vi "Model - DeInit.vi"(8 "error in (no error)":errorcluster, 11 "View Model":T1) -> (0 "error out":errorcluster)   [LabVIEW 2017]
doc: "De - initialize View Model"
uses:
  Controls/View Model.ctl
  Error Handler/Controls/Error Model.ctl
  Error Handler/Controls/Error Type.ctl
  Controls/Shared Model.ctl
  Elevator Controller/Controls/Elevator Model.ctl
  Elevator Controller/Controls/Controller Overhead.ctl
  Elevator Controller/Controls/Elevator Commands.ctl
  Configuration/Controls/Configuration Model.ctl
  Configuration/Controls/Configuration Data.ctl
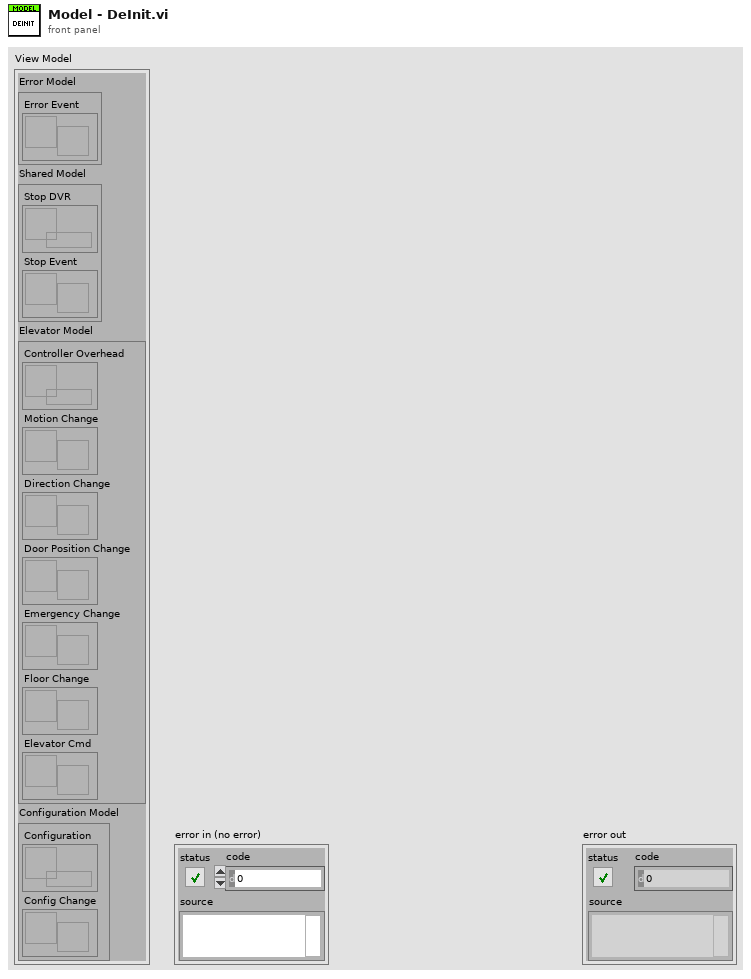
[diagram p1: front panel]
types:
  T1 = typedef "View Model.ctl" = cluster{"Error Model":T2, "Shared Model":T3, "Elevator Model":T4, "Configuration Model":T5}
  T2 = typedef "Error Model.ctl" = cluster{"Error Event":refnum<user-event>}
  T3 = typedef "Shared Model.ctl" = cluster{"Stop DVR":refnum<data-value>, "Stop Event":refnum<user-event>}
  T4 = typedef "Elevator Model.ctl" = cluster{"Controller Overhead":refnum<data-value>, "Motion Change":refnum<user-event>, "Direction Change":refnum<user-event>, "Door Position Change":refnum<user-event>, "Emergency Change":refnum<user-event>, "Floor Change":refnum<user-event>, "Elevator Cmd":refnum<user-event>}
  T5 = typedef "Configuration Model.ctl" = cluster{"Configuration":refnum<data-value>, "Config Change":refnum<user-event>}
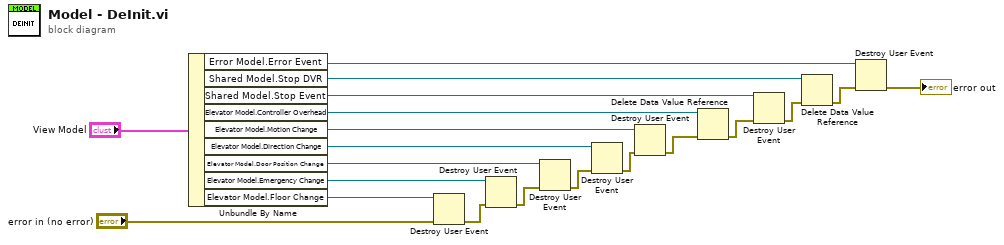
[diagram p0: block diagram]
diagram:
  n1 = Unbundle By Name("View Model") -> ("Error Model.Error Event"=w7:refnum<user-event>, "Shared Model.Stop DVR"=w8:refnum<data-value>, "Shared Model.Stop Event"=w9:refnum<user-event>, "Elevator Model.Controller Overhead"=w10:refnum<data-value>, "Elevator Model.Motion Change"=w15:refnum<user-event>, "Elevator Model.Direction Change"=w16:refnum<user-event>, "Elevator Model.Door Position Change"=w17:refnum<user-event>, "Elevator Model.Emergency Change"=w18:refnum<user-event>, "Elevator Model.Floor Change"=w19:refnum<user-event>)
  n2 = Destroy User Event(user event=w19, error in="error in (no error)") -> (error out=w14:errorcluster)
  n3 = Destroy User Event(user event=w18, error in=w14) -> (error out=w13:errorcluster)
  n4 = Destroy User Event(user event=w17, error in=w13) -> (error out=w12:errorcluster)
  n5 = Destroy User Event(user event=w16, error in=w12) -> (error out=w11:errorcluster)
  n6 = Destroy User Event(user event=w15, error in=w11) -> (error out=w6:errorcluster)
  n7 = Delete Data Value Reference(data value reference=w10, error in=w6) -> (error out=w5:errorcluster)  [unwired: 1 out]
  n8 = Destroy User Event(user event=w9, error in=w5) -> (error out=w4:errorcluster)
  n9 = Delete Data Value Reference(data value reference=w8, error in=w4) -> (error out=w3:errorcluster)  [unwired: 1 out]
  n10 = Destroy User Event(user event=w7, error in=w3) -> (error out=→"error out":errorcluster)
